vi "Read classes.vi"(9 "PythonConverter_BD in":refnum<class "PythonBDConverter.lvclass">) -> (3 "PythonConverter_BD out":refnum<class "PythonBDConverter.lvclass">, 4 "classes":variant)   [LabVIEW 2014, in "PythonBDConverter.lvclass"]
uses:
  PythonBDConverter.lvclass
  PythonBDConverter.lvclass/PythonBDConverter.ctl
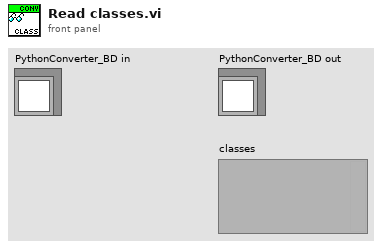
[diagram p1: front panel]
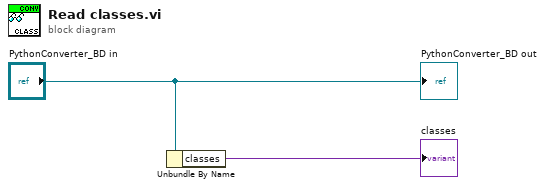
[diagram p0: block diagram]
diagram:
  n1 = Unbundle By Name("PythonConverter_BD in") -> ("classes"=→"classes":variant)
  "PythonConverter_BD out" <- "PythonConverter_BD in"
